vi "prependTopLevelNameForUpdateValueServer.vi"(10 "Array in":T1[](array[typedef]) {"New Value" format="%.2f"}, 11 "TopLevelADAMname":string) -> (3 "Array out":T1[](array[typedef]) {"New Value" format="%.2f"})   [LabVIEW 2016]
uses:
  ADAM Controls/Update_scan_value.ctl
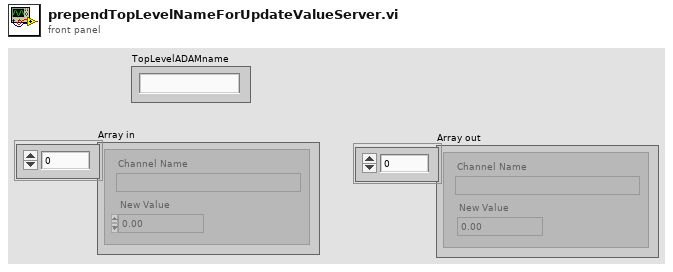
[diagram p1: front panel]
types:
  T1 = typedef "Update_scan_value.ctl" = cluster{"Channel Name":string, "New Value":dbl}
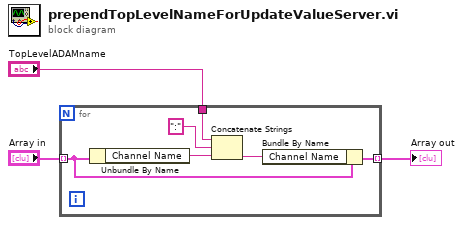
[diagram p0: block diagram]
diagram:
  n1 = for {
    tunnel: "Array in" -> [w4] mode=indexing
    tunnel: "TopLevelADAMname" -> [w8]
    tunnel: [w5] -> w2 mode=indexing
    n2 = Unbundle By Name(w4) -> ("Channel Name"=w9:string)
    n3 = Concatenate Strings(w8, ":" ("string"), w9) -> (w6:string)
    n4 = Bundle By Name(cluster=w4, "Channel Name"=w6) -> (w5:T1)
  }
  "Array out" <- w2
